vi "CreateFormatter.vi"(6 "Validate":bool=TRUE, 7 "Format":string, 8 "error in (no error)":errorcluster, 9 "Style":string, 10 "DateFormat":string, 11 "Logger in":refnum<class "Logger.lvclass">) -> (0 "error out":errorcluster, 2 "Formatter":refnum<class "Formatter.lvclass">, 3 "Logger out":refnum<class "Logger.lvclass">)   [LabVIEW 2022 SP3, in "Logger.lvlib" / "Logger.lvclass"]
uses:
  Logger.lvclass
  Logger.lvclass/Logger.ctl
  Formatter/Formatter.lvclass
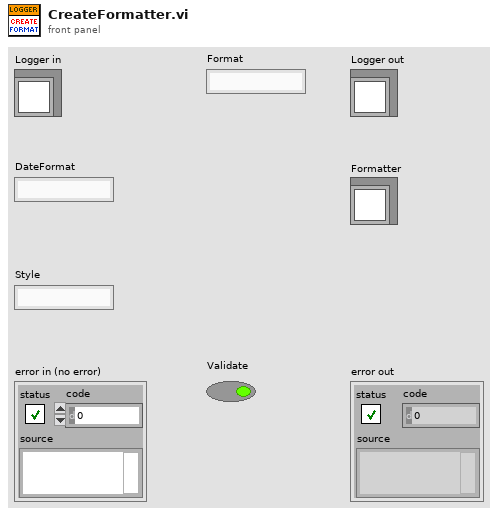
[diagram p1: front panel]
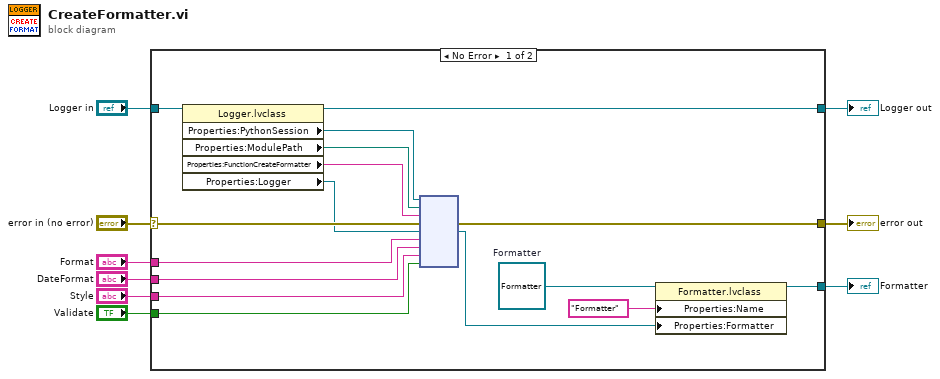
[diagram p0: block diagram]
diagram:
  n1 = case shown="No Error" "error in (no error)" {
    selector: "error in (no error)" -> [w23 w27]
    tunnel: [w14 w27] -> w5
    tunnel: [w24 w26] -> w7
    tunnel: "Logger in" -> [w25 w26]
    tunnel: "Format" -> [w18 _]
    tunnel: "DateFormat" -> [w17 _]
    tunnel: "Style" -> [w16 _]
    tunnel: "Validate" -> [w15 _]
    tunnel: [w10 _] -> w6
    frame No Error {
      w13 = refnum<class "Formatter.lvclass"> refnum  # Formatter
      n2 = property class="Logger.lvclass"(reference=w25) -> (reference out=w24:refnum<class "Logger.lvclass">, "Properties:PythonSession"=w22:refnum<k35>, "Properties:ModulePath"=w20:path, "Properties:FunctionCreateFormatter"=w21:string, "Properties:Logger"=w19:refnum<k38>)  [unwired: 1 in, 1 out]
      n3 = node(w22, w20, w21, w23, w19, w18, w17, w16, w15) -> (w14:errorcluster, w11:refnum<k38>)  [unwired: 4 in, 3 out]
      n4 = property class="Formatter.lvclass"(reference=w13, "Properties:Name"="Formatter" ("Name"), "Properties:Formatter"=w11) -> (reference out=w10:refnum<class "Formatter.lvclass">)  [unwired: 1 in, 1 out]
    }
    frame Error {
    }
  }
  "error out" <- w5
  "Logger out" <- w7
  "Formatter" <- w6
